vi "MB 2byte address.vi"(11 "Serial Parameters":T1) -> (3 "string":string)   [LabVIEW 2019]
uses:
  SerialParameters.ctl
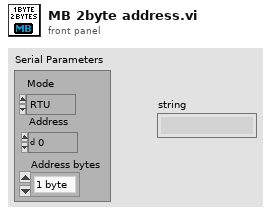
[diagram p1: front panel]
types:
  T1 = typedef "SerialParameters.ctl" = cluster{"Mode":enum16{"RTU", "ASCII"}, "Address":u16, "Address bytes":enum16{"1 byte", "2 bytes"}}
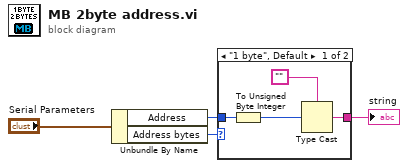
[diagram p0: block diagram]
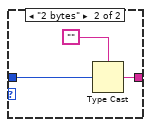
[diagram p2: hidden frame]
diagram:
  n1 = Unbundle By Name("Serial Parameters") -> ("Address"=w2:u16, "Address bytes"=w3:enum16{"1 byte", "2 bytes"})
  n2 = case shown="\"1 byte\", Default" w3 {
    tunnel: w2 -> [w8 w10]
    tunnel: [w5 w9] -> w1
    frame "1 byte", Default {
      n3 = To Unsigned Byte Integer(number=w8) -> (unsigned 8bit integer=w6:u8)
      n4 = Type Cast(type="", x=w6) -> (*(type *) &x=w5:string)
    }
    frame "2 bytes" {
      n5 = Type Cast(type="", x=w10) -> (*(type *) &x=w9:string)
    }
  }
  "string" <- w1
